vi "MoveMultiDrives.vi"(0 "Start Counter":dbl[](array[numeric]), 1 "Matched Configurations In":T2[](array[typedef]) {"Static Drive Configuration"."Indexer Mode  (FSA)" items=["Incremental", "Absolute"]; "Static Drive Configuration"."Buffer at Stop (SSH)" items=["Clear buffer", "Save and Continue"]; "Static Drive Configuration"."Buffer at Limit (SSG)" items=["Clear buffer", "Save and Continue"]; "Static Drive Configuration"."RS232 Echo Control (SSA)" items=["Echo ON", "Echo OFF"]; "Static Drive Configuration"."Reference edge of Home (OSH)" items=["CW", "CCW"]; "Static Drive Configuration"."Encoder Z for Home (OSD)" items=["Don't use", "Enable"]; "Static Drive Configuration"."Home Switch Sense (OSC)" items=["Normally Open", "Normally Closed"]; "Static Drive Configuration"."Home Position (OSB)" items=["Anywhere in Switch", "Edge of Switch"]; "Static Drive Configuration"."Limit Switch Sense (OSA)" items=["Normally Closed", "Normally Open"]; "Static Drive Configuration"."Limit Disable (LD)" items=["Both Enabled", "CW Disabled", "CCW Disabled", "Both Disabled"]; "Static Drive Configuration"."Stall Detect (FSH)" items=["Disable", "Enable"]; "Static Drive Configuration"."OP2 in Deadband (FSG)" items=["Don't Use", "ACTIVATE"]; "Static Drive Configuration"."Stop on Trigger 3 (FSF)" items=["Ignore", "STOP!"]; "Static Drive Configuration"."Activate OP1 on stall (FSE)" items=["Do not Activate", "ACTIVATE!"]; "Static Drive Configuration"."Stop on Stall (FSD)" items=["Continue", "STOP"]; "Static Drive Configuration"."Position Maintenance (FSC)" items=["Disabled", "Enabled"]; "Static Drive Configuration"."Step Mode  (FSB)" items=["Motor", "Encoder"]; "Static Drive Configuration"."Encoder Resolution (ER)" min=1 max=50000; "Static Drive Configuration"."Dead Band Window (DW)" min=0 max=999999999; "Static Drive Configuration"."Dead Band (DB)" min=0 max=999999999; "Static Drive Configuration"."Correction Gain % (CG)" items=["n/a", "12.5", "25", "37.5", "50", "62.5", "75", "87.5", "100"]; "Channel Properties"."Current Pos" format="%.2f"; "Channel Properties"."Backlash/Eng units" format="%.2f"; "Channel Properties"."Pulses/rev" format="%.2f"; "Channel Properties"."Pos Tolerance" format="%.2f"; "Channel Properties"."Pulses/unit" format="%.2f"; "Channel Properties"."Acc. Min" format="%.2f"; "Channel Properties"."Acc. Max" format="%.2f"; "Channel Properties"."Vel. Min" format="%.2f"; "Channel Properties"."Vel. Max" format="%.2f"; "Channel Properties"."Acc. Default" format="%.2f"; "Channel Properties"."Vel. Default" format="%.2f"}, 2 "GoTo Array (pulse position some channels)":T5[](array[typedef]) {"Acceleration" format="%.2f"; "Velocity" format="%.2f"; "Go To Position" step=100000.0}, 3 "Final move":bool, 4 "Predicted Move Time":dbl format="%.2f") -> (5 "Error string":string, 6 "Stop Pressed?":bool, 7 "Matched Configurations Out":T2[](array[typedef]) {"Static Drive Configuration"."Indexer Mode  (FSA)" items=["Incremental", "Absolute"]; "Static Drive Configuration"."Buffer at Stop (SSH)" items=["Clear buffer", "Save and Continue"]; "Static Drive Configuration"."Buffer at Limit (SSG)" items=["Clear buffer", "Save and Continue"]; "Static Drive Configuration"."RS232 Echo Control (SSA)" items=["Echo ON", "Echo OFF"]; "Static Drive Configuration"."Reference edge of Home (OSH)" items=["CW", "CCW"]; "Static Drive Configuration"."Encoder Z for Home (OSD)" items=["Don't use", "Enable"]; "Static Drive Configuration"."Home Switch Sense (OSC)" items=["Normally Open", "Normally Closed"]; "Static Drive Configuration"."Home Position (OSB)" items=["Anywhere in Switch", "Edge of Switch"]; "Static Drive Configuration"."Limit Switch Sense (OSA)" items=["Normally Closed", "Normally Open"]; "Static Drive Configuration"."Limit Disable (LD)" items=["Both Enabled", "CW Disabled", "CCW Disabled", "Both Disabled"]; "Static Drive Configuration"."Stall Detect (FSH)" items=["Disable", "Enable"]; "Static Drive Configuration"."OP2 in Deadband (FSG)" items=["Don't Use", "ACTIVATE"]; "Static Drive Configuration"."Stop on Trigger 3 (FSF)" items=["Ignore", "STOP!"]; "Static Drive Configuration"."Activate OP1 on stall (FSE)" items=["Do not Activate", "ACTIVATE!"]; "Static Drive Configuration"."Stop on Stall (FSD)" items=["Continue", "STOP"]; "Static Drive Configuration"."Position Maintenance (FSC)" items=["Disabled", "Enabled"]; "Static Drive Configuration"."Step Mode  (FSB)" items=["Motor", "Encoder"]; "Static Drive Configuration"."Encoder Resolution (ER)" min=1 max=50000; "Static Drive Configuration"."Dead Band Window (DW)" min=0 max=999999999; "Static Drive Configuration"."Dead Band (DB)" min=0 max=999999999; "Static Drive Configuration"."Correction Gain % (CG)" items=["n/a", "12.5", "25", "37.5", "50", "62.5", "75", "87.5", "100"]; "Channel Properties"."Current Pos" format="%.2f"; "Channel Properties"."Backlash/Eng units" format="%.2f"; "Channel Properties"."Pulses/rev" format="%.2f"; "Channel Properties"."Pos Tolerance" format="%.2f"; "Channel Properties"."Pulses/unit" format="%.2f"; "Channel Properties"."Acc. Min" format="%.2f"; "Channel Properties"."Acc. Max" format="%.2f"; "Channel Properties"."Vel. Min" format="%.2f"; "Channel Properties"."Vel. Max" format="%.2f"; "Channel Properties"."Acc. Default" format="%.2f"; "Channel Properties"."Vel. Default" format="%.2f"})   [LabVIEW 2012]
uses:
  ~subVIs/DriveClusterLower.ctl
  ~subVIs/AxisConfigCluster.ctl
  ~subVIs/DriveProperties.ctl
  ~subVIs/DriveStaticConfig.ctl
  ~subVIs/DriveStatus.ctl
  ~subVIs/GenericDriveCommand.ctl
  ~subVIs/DriveConfigGlobal.vi
  Anemometry/Anemometry Sub Vis/Globals/Trav_pos_global.vi
panel:
  out "x*y":dbl
  out "Move On Track?":bool
  out "Live Position":dbl[](array[numeric]) format="%.2f"
  out "Server copy Location":path
  out "Log File":path
  out "Move Terminated on Timeout":bool
  in  "Axis info cluster":T1
  out "Start Time":dbl format="%.2f"
  out "Running":bool
  out "Bar2":dbl(slide)=2.0 scale=-599243.8..-600063.0
  out "Bar1":dbl(slide)=2.0 scale=233922.756..233952.0
  out "Bar0":dbl(slide)=2.0 scale=322356.2..321537.0
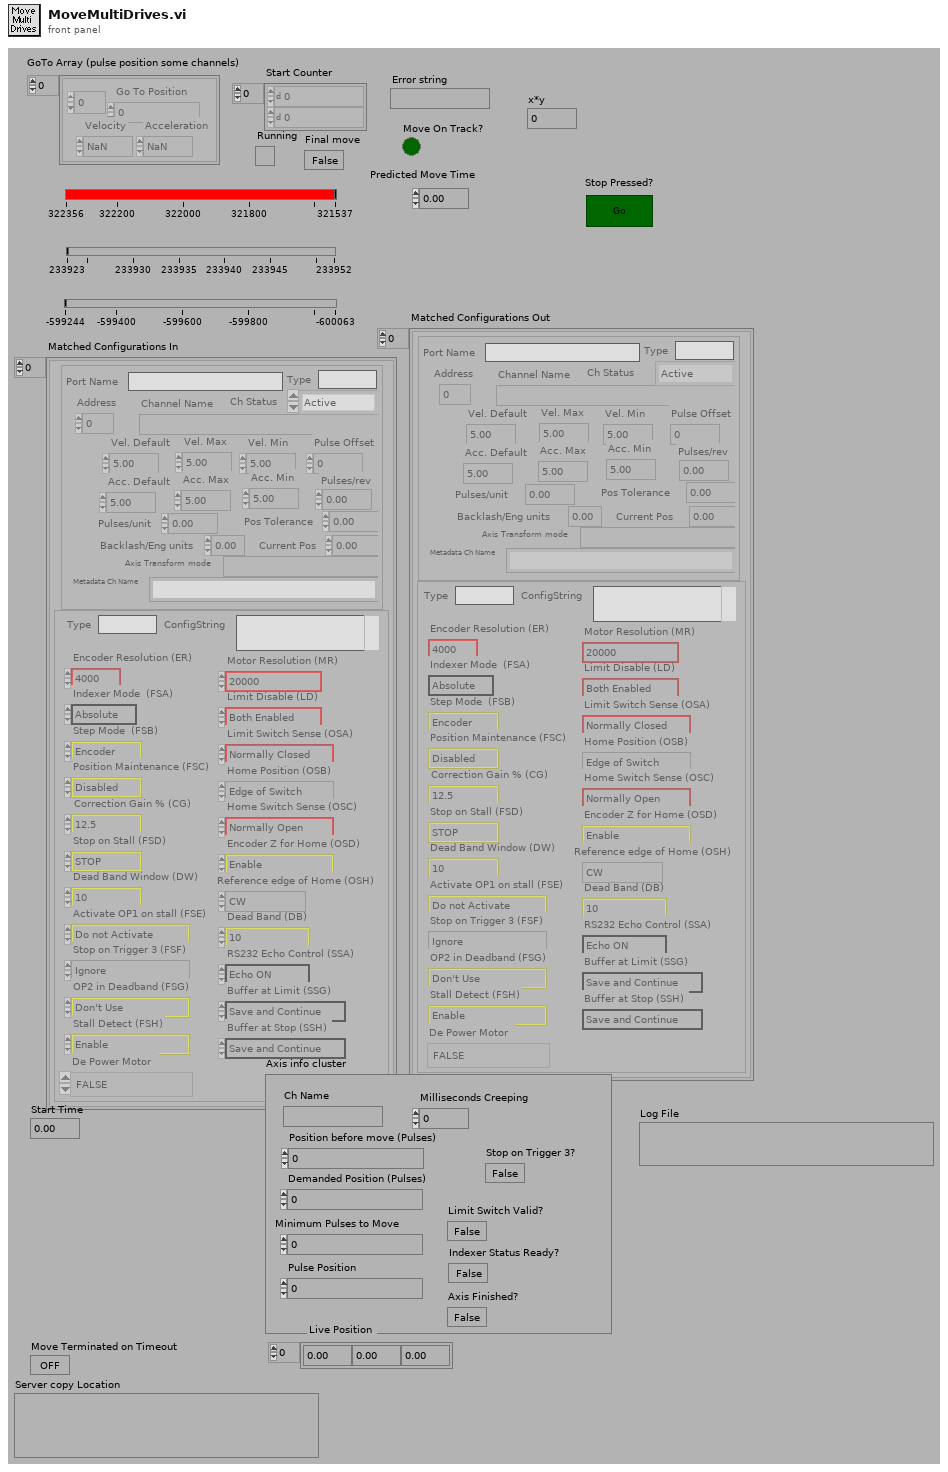
[diagram p1: front panel]
types:
  T1 = typedef "DriveStatus.ctl" = cluster{"Ch Name":string, "Position before move (Pulses)":dbl, "Demanded Position (Pulses)":dbl, "Minimum Pulses to Move":dbl, "Pulse Position":dbl, "Indexer Status Ready?":bool, "Axis Finished?":bool, "Limit Switch Valid?":bool, "Milliseconds Creeping":u32, "Stop on Trigger 3?":bool}
  T2 = typedef "AxisConfigCluster.ctl" = cluster{"Channel Properties":T3, "Static Drive Configuration":T4}
  T3 = typedef "DriveProperties.ctl" = cluster{"Channel Name":string, "Vel. Default":dbl, "Acc. Default":dbl, "Vel. Max":dbl, "Vel. Min":dbl, "Acc. Max":dbl, "Acc. Min":dbl, "Pulses/unit":dbl, "Address":u8, "Pulse Offset":i32, "Pos Tolerance":dbl, "Pulses/rev":dbl, "Backlash/Eng units":dbl, "Current Pos":dbl, "Ch Status":enum16{"Active", "Offline", "Simulate"}, "Port Name":string, "Axis Transform mode":string, "Metadata Ch Name":string, "Type":string}
  T4 = typedef "DriveStaticConfig.ctl" = cluster{"Correction Gain % (CG)":u16, "Dead Band (DB)":i32, "Dead Band Window (DW)":i32, "Encoder Resolution (ER)":i32, "Step Mode  (FSB)":u16, "Position Maintenance (FSC)":u16, "Stop on Stall (FSD)":u16, "Activate OP1 on stall (FSE)":u16, "Stop on Trigger 3 (FSF)":u16, "OP2 in Deadband (FSG)":u16, "Stall Detect (FSH)":u16, "Limit Disable (LD)":u16, "Motor Resolution (MR)":enum16{"200", "400", "1000", "2000", "4000", "5000", "10000", "12800", "18000", "20000", "21600", "25000", "25400", "25600", "36000", "50000", "278528", "425984", "507904", "614400", "655360", "819200", "1024000"}, "Limit Switch Sense (OSA)":u16, "Home Position (OSB)":u16, "Home Switch Sense (OSC)":u16, "Encoder Z for Home (OSD)":u16, "Reference edge of Home (OSH)":u16, "RS232 Echo Control (SSA)":u16, "Buffer at Limit (SSG)":u16, "Buffer at Stop (SSH)":u16, "Indexer Mode  (FSA)":u16, "Type":string, "ConfigString":string, "De Power Motor":enum16{"TRUE", "FALSE"}}
  T5 = typedef "DriveClusterLower.ctl" = cluster{"Go To Position":dbl, "Velocity":dbl, "Acceleration":dbl, "Address":u8}
  T6 = typedef "GenericDriveCommand.ctl" = string
  T7 = cluster{"GenericDriveCommand":T6, "Go To Position":dbl}
  T8 = cluster{"GenericDriveCommand":T6, "Acceleration":dbl}
  T9 = cluster{"GenericDriveCommand":T6, "Acceleration":dbl}[]
  T10 = enum16{"A-    Acceleration (rps)", "B-    Buffer Status", "C-    Continue", "CG-  Correction Gain", "CR-  Cariage Return", "D-    Distance (pulses)", "DB-  Dead Band (encoder steps)", "DW- Deadband Window (encoder steps)", "E-    Enable Communications", "ER-  Encoder Resolution (steps/rev)", "F-    Disable Communications", "FS-  Encoder Functions Report", "FSA- Incremental/Absolute (0/1)", "FSB- Motor/Encoder Step Mode (0/1)", "FSC- Enable/Disable Position Maint. (1/0)", "FSD- Stop/Continue on Stall (1/0)", "FSE- Activate o/p1 on Stall (1/0)", "FSF- Stop Motion on Trig3 (1/0)", "FSG- Activate o/p2 in Deadband (1/0)", "FSH- Enable Stall Detect (1/0)", "G- Go", "GH- Go Home and Zero (+/-V)", "^H- Delete ", "H- Direction Reverse/CCW/CW (0,1,2)", "IS- Input Status", "K- Kill", "L- Loop (n)", "LD- Limit DISABLE (0-none,1-CW,2-CCW,3-Both)", "LF- Line Feed", "MC- Mode Continuous", "MN- Mode Normal", "MPA- Motor Postion Absolute", "MPI- Motor Position Incremental", "MR- Motor Resolution (Drive Steps/rev)", "N- End of Loop", "O- Output (00,01,10,11)", "OS- Report Homing Setup", "OSA- NO/NC Limits (1/0)", "OSB- Back Up to Home/Edge? (0/1)", "OSC- NO/NC Home Switch (1/0)", "OSD- Enable Encoder Z for Home (0/1)", "OSH- Reference Edge for Home CW/CCW (0/1)", "PR- Report ABSOLUTE Position", "PS- Pause until Continue", "PX- Report Absolute ENCODER Position", "PZ- Zero Absolute Counter", "\"- Quote (17 ASCII +Space)", "Q- Enter/Exit Velocity Profiling (1/0)", "R- Request Indexer Status", "RA- Report Limit Switch Status", "RB- Report Loop, Pause, Shutdown, Trigger Status", "RC- Report Closed Loop Status", "RM- Velocity Streaming Rate Multiplier (000-FFF)", "RV- Report Revision Level", "S- Controlled Stop", "SN- Debounce (1-1000ms)", "SS- Report Software Switch Status", "SSA- Disable RS232 Echo (1/0)", "SSG- Clear/Save Command Buffer on Limit (0/1)", "SSH- Clear/Save Command Buffer on Stop (0/1)", "ST- Shutdown (1/0)", "SV- Servoing Setting (0,1,2,3)", "T- Time Delay (0.01-99999.99)", "TR- Wait for Trigger High/Low/Ignore (1/0/X)", "TS- Report Trigger Status", "U- Pause after Move Until Continue", "V- Velocity (0.01-50.00 revs/sec)", "W1- Report Relative Position <Signed Binary>", "W3- Report Relative Position <Hexadecimal>", "Y- Abort Loop at N", "Z-    Reset to Defaults", "#-    Disable/Set Soft Addresses (0/1-255)"}
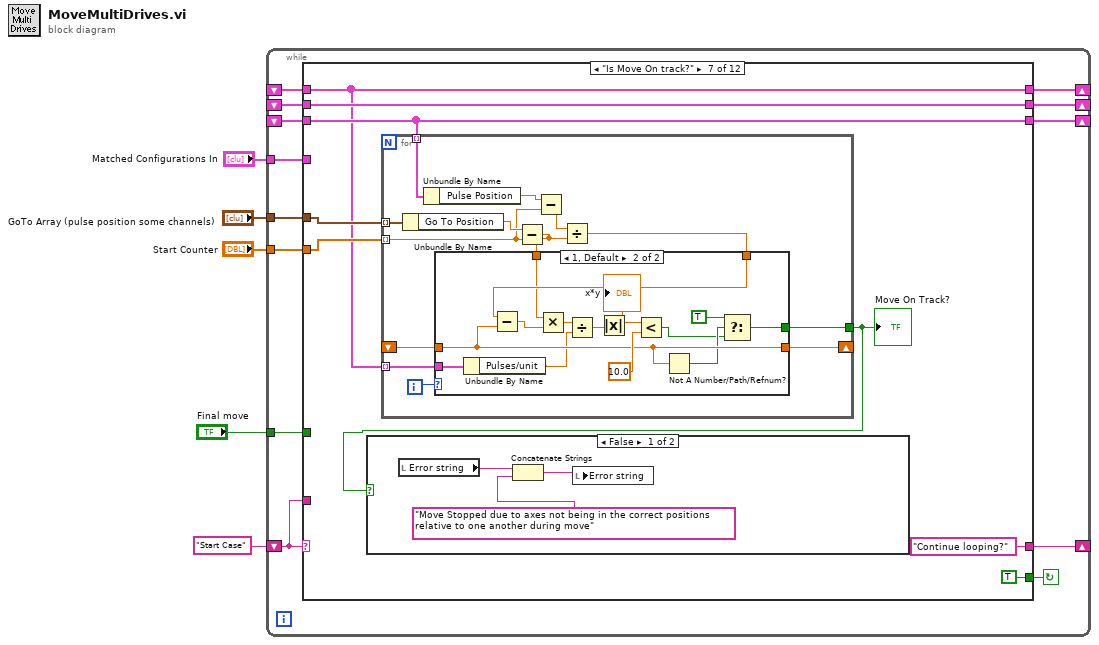
[diagram p0: block diagram]
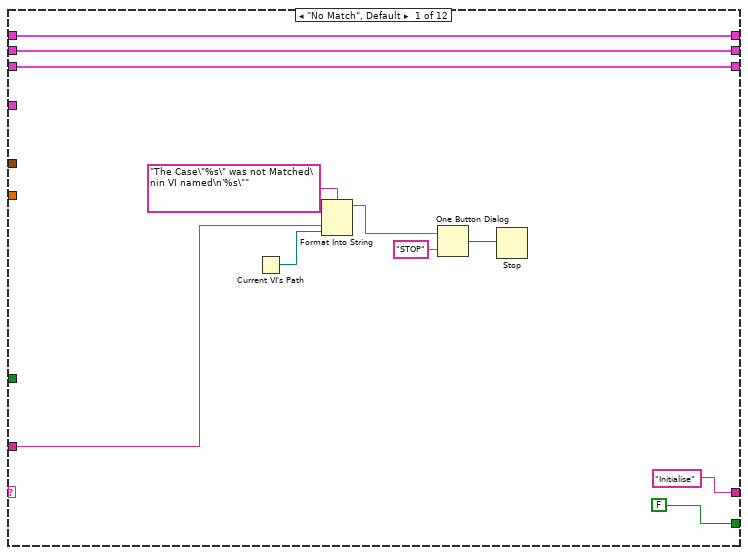
[diagram p2: hidden frame]
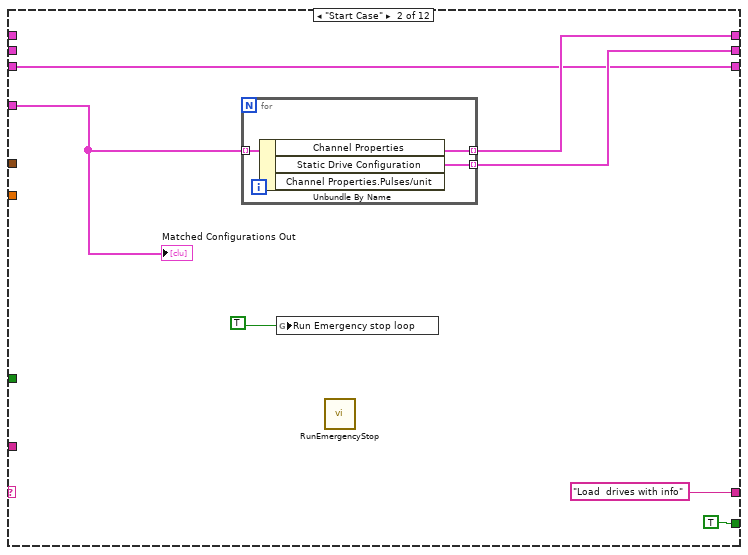
[diagram p3: hidden frame]
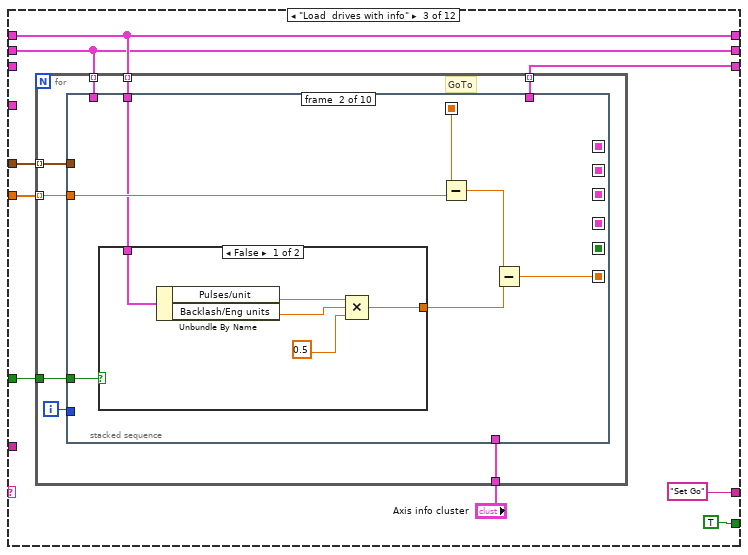
[diagram p4: hidden frame]
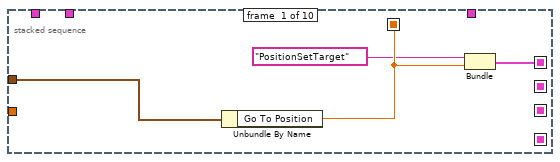
[diagram p5: hidden frame]
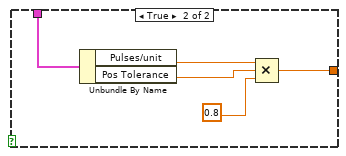
[diagram p6: hidden frame]
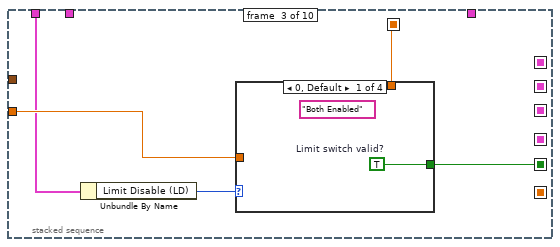
[diagram p7: hidden frame]
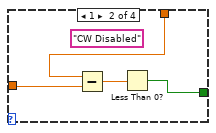
[diagram p8: hidden frame]
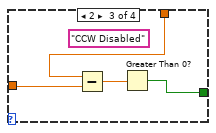
[diagram p9: hidden frame]
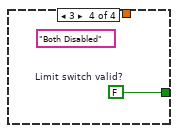
[diagram p10: hidden frame]
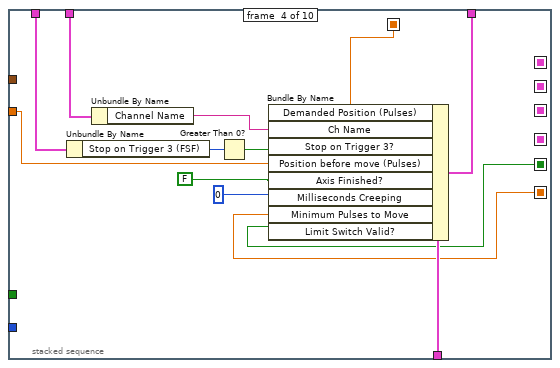
[diagram p11: hidden frame]
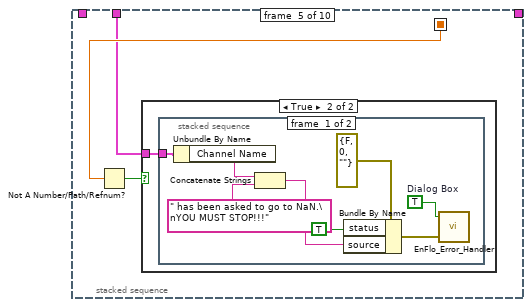
[diagram p12: hidden frame]
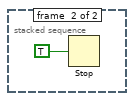
[diagram p14: hidden frame]
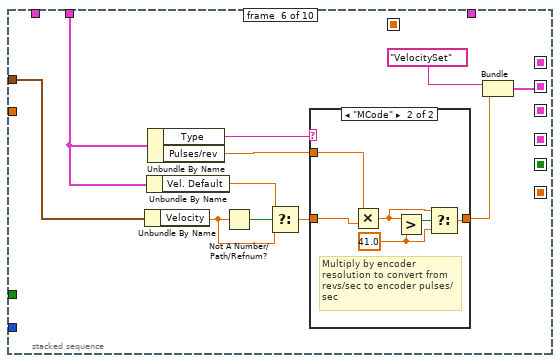
[diagram p15: hidden frame]
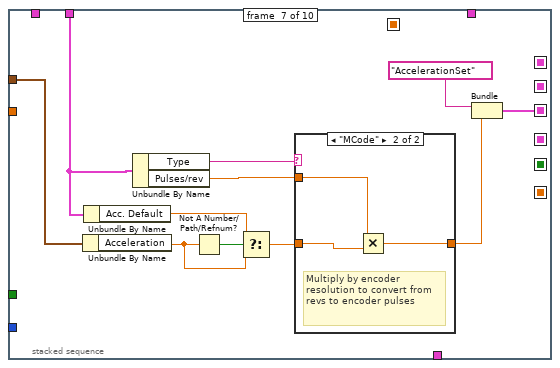
[diagram p17: hidden frame]
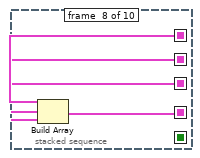
[diagram p19: hidden frame]
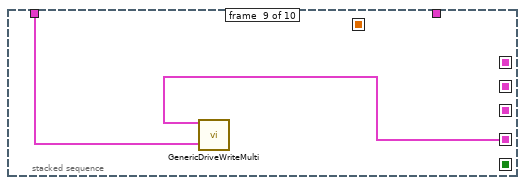
[diagram p20: hidden frame]
diagram:
  n1 = while {
    shift-left: _ -> [w7]
    shift-right: [w6] -> _
    tunnel: "Final move" -> [w8]
    tunnel: "Start Counter" -> [w9]
    tunnel: "GoTo Array (pulse position some channels)" -> [w10]
    tunnel: "Matched Configurations In" -> [w15]
    shift-left: _ -> [w11]
    shift-right: [w13] -> _
    shift-left: _ -> [w12]
    shift-right: [w14] -> _
    shift-left: "Start Case" -> [w16]
    shift-right: [w17] -> _
    stop <- w18 continue-if-true
    n2 = case shown="\"Is Move On track?\"" w16 {
      tunnel: [FALSE TRUE TRUE TRUE TRUE TRUE TRUE TRUE TRUE TRUE TRUE FALSE] -> w18
      tunnel: ["Initialise" "Load  drives with info" "Set Go" "Record Time" "Check status of axis" "Is Move On track?" "Continue looping?" w299 "Does Log file Exist" w345 "Write to Log file" "End"] -> w17
      tunnel: w16 -> [w24 _ _ _ _ _ _ _ _ _ _ _]
      tunnel: w15 -> [_ w30 _ w181 _ _ _ _ _ _ _ _]
      tunnel: [w21 w33 w45 w185 w196 w203 w256 w318 w326 w350 w371 w398] -> w14
      tunnel: [w20 w32 w42 w184 w195 w204 w261 w317 w325 w349 w370 w397] -> w13
      tunnel: w12 -> [w21 _ w45 w185 w196 w203 w256 w318 w326 w350 w371 w398]
      tunnel: w11 -> [w20 _ w42 w184 w195 w204 w261 w317 w325 w349 w370 w397]
      tunnel: w10 -> [_ _ w46 _ _ _ w263 _ _ _ _ _]
      tunnel: w9 -> [_ _ w44 _ _ _ w262 _ _ _ _ _]
      tunnel: w8 -> [_ _ w43 _ _ _ _ _ _ _ _ _]
      tunnel: [w19 w31 w40 w182 w193 w200 w260 w304 w324 w348 w369 w395] -> w6
      tunnel: w7 -> [w19 w31 _ w182 w193 w201 w260 w304 w324 w348 w369 w395]
      frame "No Match", Default {
        n3 = Current VI's Path() -> (path=w23:path)
        n4 = Format Into String(format string="The Case\"%s\" was not Matched\nin VI named\n'%s\"" ("Format String"), w24, w23) -> (resulting string=w27:string)  [unwired: 2 in, 1 out]
        n5 = One Button Dialog(message=w27, button name ("OK")="STOP") -> (true=w25:bool)
        n6 = Stop(stop? (T)=w25) -> ()
      }
      frame "Start Case" {
        n7 = for {
          tunnel: w30 -> [w39] mode=indexing
          tunnel: [w38] -> w33 mode=indexing
          tunnel: [w37] -> w32 mode=indexing
          n8 = Unbundle By Name(w39) -> ("Channel Properties"=w38:T3, "Static Drive Configuration"=w37:T4)  [unwired: 1 out]
        }
        n9 = global write "DriveConfigGlobal.vi" "Run Emergency stop loop"(TRUE) -> ()
        n10 = call "RunEmergencyStop.vi"() -> ()  [unwired: 1 in, 7 out]
        "Matched Configurations Out" <- w30
      }
      frame "Load  drives with info" {
        n11 = for {
          tunnel: w46 -> [w55] mode=indexing
          tunnel: w45 -> [w54] mode=indexing
          tunnel: w44 -> [w53] mode=indexing
          tunnel: w43 -> [w52]
          tunnel: w42 -> [w51] mode=indexing
          tunnel: "Axis info cluster" -> [w50]
          tunnel: [w49] -> w40 mode=indexing
          i -> [w56]
          # "GoTo"
          n12 = stacked-sequence {
            seq-local: [w59 _ _ _ _ _ _ _ _ _] -> [_ w67 w81 w96 w108 _ _ _ _ w163]
            seq-local: [w58 _ _ _ _ _ _ _ _ _] -> [_ _ _ _ _ _ _ w155 _ _]
            seq-local: [_ _ _ _ _ w125 _ _ _ _] -> [_ _ _ _ _ _ _ w154 _ _]
            seq-local: [_ _ _ _ _ _ w143 _ _ _] -> [_ _ _ _ _ _ _ w153 _ _]
            seq-local: [_ _ _ _ _ _ _ w152 _ _] -> [_ _ _ _ _ _ _ _ w157 _]
            seq-local: [_ w62 _ _ _ _ _ _ _ _] -> [_ _ _ w103 _ _ _ _ _ _]
            seq-local: [_ _ w78 _ _ _ _ _ _ _] -> [_ _ _ w101 _ _ _ _ _ _]
            tunnel: w55 -> [w60 _ _ _ _ w129 w147 _ _ _]
            tunnel: w56 -> [_ _ _ _ _ _ _ _ _ w164]
            tunnel: w52 -> [_ w65 _ _ _ _ _ _ _ _]
            tunnel: w54 -> [_ w63 _ w105 w106 w123 w141 _ w156 _]
            tunnel: w53 -> [_ w64 w80 w98 _ _ _ _ _ w162]
            tunnel: w51 -> [_ _ w79 w100 _ _ _ _ _ _]
            tunnel: w50 -> [_ _ _ w104 _ _ _ _ _ _]
            tunnel: [_ _ _ w102 _ _ _ _ _ _] -> w49
            frame #0 {
              n13 = Unbundle By Name(w60) -> ("Go To Position"=w59:dbl)
              n14 = Bundle("GenericDriveCommand"=T6 "PositionSetTarget", "Go To Position"=w59) -> (w58:T7)  [unwired: 1 out]
            }
            frame #1 {
              n15 = case shown="False" w65 {
                tunnel: w63 -> [w72 w77]
                tunnel: [w68 w73] -> w66
                frame False {
                  n16 = Unbundle By Name(w72) -> ("Pulses/unit"=w71:dbl, "Backlash/Eng units"=w70:dbl)
                  n17 = Compound Arithmetic op=MULTIPLY(w71, w70, 0.5) -> (w68:dbl)
                }
                frame True {
                  n18 = Unbundle By Name(w77) -> ("Pulses/unit"=w76:dbl, "Pos Tolerance"=w75:dbl)
                  n19 = Compound Arithmetic op=MULTIPLY(w76, w75, 0.8) -> (w73:dbl)
                }
              }
              n20 = Subtract(x=w67, y=w64) -> (x-y=w61:dbl)
              n21 = Subtract(x=w61, y=w66) -> (x-y=w62:dbl)
            }
            frame #2 {
              n22 = Unbundle By Name(w79) -> ("Limit Disable (LD)"=w82:u16)
              n23 = case shown="0, Default" w82 {
                tunnel: [w83 w84 w88 w92] -> w78
                tunnel: w80 -> [_ w86 w90 _]
                tunnel: w81 -> [_ w87 w91 _]
                frame 0, Default {
                  w83 = TRUE  # Limit switch valid?
                  (unwired) "Both Enabled"
                }
                frame 1 {
                  (unwired) "CW Disabled"
                  n24 = Subtract(x=w87, y=w86) -> (x-y=w85:dbl)
                  n25 = Less Than 0?(x=w85) -> (x < 0?=w84:bool)
                }
                frame 2 {
                  (unwired) "CCW Disabled"
                  n26 = Subtract(x=w91, y=w90) -> (x-y=w89:dbl)
                  n27 = Greater Than 0?(x=w89) -> (x > 0?=w88:bool)
                }
                frame 3 {
                  (unwired) "Both Disabled"
                  w92 = FALSE  # Limit switch valid?
                }
              }
            }
            frame #3 {
              n28 = Unbundle By Name(w100) -> ("Stop on Trigger 3 (FSF)"=w99:u16)
              n29 = Unbundle By Name(w105) -> ("Channel Name"=w97:string)
              n30 = Greater Than 0?(x=w99) -> (x > 0?=w95:bool)
              n31 = Bundle By Name(cluster=w104, "Demanded Position (Pulses)"=w96, "Ch Name"=w97, "Stop on Trigger 3?"=w95, "Position before move (Pulses)"=w98, "Axis Finished?"=FALSE ("Bundle Element"), "Milliseconds Creeping"=u32 0 ("Bundle Element"), "Minimum Pulses to Move"=w103, "Limit Switch Valid?"=w101) -> (w102:T1)
            }
            frame #4 {
              n32 = Not A Number/Path/Refnum?(number/path/refnum=w108) -> (NaN/Path/Refnum?=w107:bool)
              n33 = case shown="True" w107 {
                tunnel: w106 -> [_ w109]
                frame False {
                }
                frame True {
                  n34 = stacked-sequence {
                    tunnel: w109 -> [w117 _]
                    frame #0 {
                      w110 = TRUE  # Dialog Box
                      n35 = Unbundle By Name(w117) -> ("Channel Name"=w113:string)
                      n36 = Concatenate Strings(w113, " has been asked to go to NaN.\nYOU MUST STOP!!!") -> (w111:string)
                      n37 = Bundle By Name(cluster=errorcluster {"status"=FALSE, "code"=0, "source"=""} ("error in (no error)"), "status"=TRUE ("Bundle Element"), "source"=w111) -> (w115:errorcluster)
                      n38 = call "EnFlo_Error_Handler.vi"("error in (no error)"=w115, "Dialog Box (T)"=w110) -> ()  [unwired: 1 in, 3 out]
                    }
                    frame #1 {
                      n39 = Stop(stop? (T)=TRUE) -> ()
                    }
                  }
                }
              }
            }
            frame #5 {
              n40 = Unbundle By Name(w129) -> ("Velocity"=w126:dbl)
              n41 = Unbundle By Name(w123) -> ("Vel. Default"=w127:dbl)
              n42 = Unbundle By Name(w123) -> ("Type"=w122:string, "Pulses/rev"=w120:dbl)
              n43 = Not A Number/Path/Refnum?(number/path/refnum=w126) -> (NaN/Path/Refnum?=w128:bool)
              n44 = Select(t=w127, s=w128, f=w126) -> (s? t:f=w121:dbl)
              n45 = case shown="\"MCode\"" w122 {
                tunnel: w121 -> [w130 w131]
                tunnel: w120 -> [_ w136]
                tunnel: [w130 w135] -> w119
                frame "ParkerX", Default {
                }
                frame "MCode" {
                  w132 = 41.0 ("y")
                  # "Multiply by encoder resolution to convert from revs/sec to encoder pulses/sec"
                  n46 = Multiply(x=w136, y=w131) -> (x*y=w133:dbl)
                  n47 = Greater?(x=w133, y=w132) -> (0:w134:bool)
                  n48 = Select(t=w133, s=w134, f=w132) -> (s? t:f=w135:dbl)
                }
              }
              n49 = Bundle("GenericDriveCommand"=T6 "VelocitySet", "y"=w119) -> (w125:cluster{"GenericDriveCommand":T6, "y":dbl})  [unwired: 1 out]
            }
            frame #6 {
              n50 = Unbundle By Name(w147) -> ("Acceleration"=w144:dbl)
              n51 = Unbundle By Name(w141) -> ("Acc. Default"=w145:dbl)
              n52 = Unbundle By Name(w141) -> ("Type"=w140:string, "Pulses/rev"=w139:dbl)
              n53 = Not A Number/Path/Refnum?(number/path/refnum=w144) -> (NaN/Path/Refnum?=w146:bool)
              n54 = Select(t=w145, s=w146, f=w144) -> (s? t:f=w138:dbl)
              n55 = case shown="\"MCode\"" w140 {
                tunnel: w138 -> [w148 w151]
                tunnel: w139 -> [_ w150]
                tunnel: [w148 w149] -> w137
                frame "ParkerX", Default {
                }
                frame "MCode" {
                  # "Multiply by encoder resolution to convert from revs to encoder pulses"
                  n56 = Multiply(x=w150, y=w151) -> (x*y=w149:dbl)
                }
              }
              n57 = Bundle("GenericDriveCommand"=T6 "AccelerationSet", "Acceleration"=w137) -> (w143:T8)  [unwired: 1 out]
            }
            frame #7 {
              n58 = Build Array(w155, w154, w153) -> (w152:T9)
            }
            frame #8 {
              n59 = call "GenericDriveWriteMulti.vi"("Channel Description"=w156, "Array Constant"=w157) -> ()  [unwired: 1 out]
            }
            frame #9 {
              n60 = Less?(x=w163, y=w162) -> (x < y?=w161:bool)
              n61 = Max & Min(x=w163, y=w162) -> (max(x,y)=w166:dbl, min(x,y)=w165:dbl)
              n62 = Select(t=2, s=w161, f=1 ("Fill Style")) -> (s? t:f=w158:i32)
              n63 = case shown="1" w164 {
                tunnel: w166 -> [w170 w174 w178]
                tunnel: w165 -> [w169 w173 w177]
                tunnel: w161 -> [w168 w172 w176]
                tunnel: w158 -> [w167 w171 w175]
                frame 0, Default {
                  n64 = property on="Bar0" class="Slide (strict)"("Scale.Range:Maximum"=w170, "Scale.Range:Minimum"=w169, "Scale.Flipped"=w168, "Fill Style"=w167) -> ()  [unwired: 2 in, 2 out]
                }
                frame 1 {
                  n65 = property on="Bar1" class="Slide (strict)"("Scale.Range:Maximum"=w174, "Scale.Range:Minimum"=w173, "Scale.Flipped"=w172, "Fill Style"=w171) -> ()  [unwired: 2 in, 2 out]
                }
                frame 2 {
                  n66 = property on="Bar2" class="Slide (strict)"("Scale.Range:Maximum"=w178, "Scale.Range:Minimum"=w177, "Scale.Flipped"=w176, "Fill Style"=w175) -> ()  [unwired: 2 in, 2 out]
                }
              }
            }
          }
        }
      }
      frame "Set Go" {
        n67 = call "GetActivePortNames.vi"("Matched Configurations In"=w181) -> ("Port Name Array"=w180:string[], "Drive Type Array"=w179:string[])
        n68 = for {
          tunnel: w180 -> [w191] mode=indexing
          tunnel: "Global" -> [w190]
          tunnel: w179 -> [w189] mode=indexing
          n69 = call "GenericDriveIO.vi"("GenericDriveCommand"=T6 "GoNow", "Channel Name"=w190, "Type"=w189, "Port Name"=w191) -> ()  [unwired: 2 in, 6 out]
        }
      }
      frame "Record Time" {
        n70 = Get Date/Time In Seconds() -> (seconds since 1Jan1904=w192:timestamp)
        n71 = To Double Precision Float(number=w192) -> (double precision float=→"Start Time":dbl)
      }
      frame "Check status of axis" {
        (unwired) "Global"
        n72 = for {
          shift-right: [w210] -> w199
          shift-left: "" -> [w212]
          tunnel: w203 -> [w211] mode=indexing
          tunnel: w201 -> [w208] mode=indexing
          tunnel: [w207] -> w200 mode=indexing
          i -> [w213]
          n73 = Unbundle By Name(w208) -> ("Axis Finished?"=w209:bool)
          n74 = case shown="False" w209 {
            tunnel: w213 -> [w235 _]
            tunnel: w212 -> [w234 w255]
            tunnel: w211 -> [w229 _]
            tunnel: [w232 w255] -> w210
            tunnel: w208 -> [w231 w254]
            tunnel: [w230 w254] -> w207
            frame False {
              n75 = Unbundle By Name(w229) -> ("Channel Name"=w224:string, "Pulses/unit"=w228:dbl, "Pulse Offset"=w225:i32)
              n76 = call "CheckDriveStatus.vi"("Channel Properties"=w229, "Axis info cluster"=w231) -> ("Error string"=w233:string, "Axis info cluster Out"=w230:T1)
              n77 = Unbundle By Name(w230) -> ("Pulse Position"=w214:dbl)
              n78 = global read "Trav_pos_global.vi" "Live Position"() -> (w216:dbl[])
              n79 = Match Pattern(string=w224, regular expression=":") -> (before substring=w220:string, after substring=w219:string)  [unwired: 1 in, 2 out]
              n80 = Match Pattern(string=w219, regular expression=":") -> (after substring=w218:string)  [unwired: 1 in, 3 out]
              n81 = Add(x=w225, y=w214) -> (x+y=w226:dbl)
              n82 = Divide(x=w226, y=w228) -> (x/y=w217:dbl)
              n83 = case shown="\"Z\", Default" w218 {
                tunnel: w217 -> [w237 w242 w250]
                tunnel: w216 -> [w239 w245 w249]
                tunnel: [w236 w241 w246] -> w215
                frame "Y" {
                  n84 = Index Array(array=w239) -> (element #1=w238:dbl, element #3=w240:dbl)  [unwired: 3 in, 1 out]
                  n85 = Build Array(w238, w237, w240) -> (w236:dbl[])
                }
                frame "X" {
                  n86 = Index Array(array=w245) -> (element #2=w243:dbl, element #3=w244:dbl)  [unwired: 3 in, 1 out]
                  n87 = Build Array(w242, w243, w244) -> (w241:dbl[])
                }
                frame "Z", Default {
                  n88 = Index Array(array=w249) -> (element #1=w248:dbl, element #2=w247:dbl)  [unwired: 2 in]
                  n89 = Build Array(w248, w247, w250) -> (w246:dbl[])
                }
              }
              n90 = call "Coordinate_transforms.vi"("Traverse Name"=w220, "Input"=w215, "Mode"=enum16{"XYZ to Channel", "Channel to XYZ"}."Channel to XYZ") -> ("Output"=w222:dbl[])
              "Live Position" <- w222
              n91 = Concatenate Strings(w234, w233) -> (w232:string)
              n92 = case shown="2" w235 {
                tunnel: w214 -> [w251 w252 w253]
                frame 0, Default {
                  "Bar0" <- w251
                }
                frame 1 {
                  "Bar1" <- w252
                }
                frame 2 {
                  "Bar2" <- w253
                }
              }
              n93 = global write "Trav_pos_global.vi" "Live Position"(w222) -> ()
            }
            frame True {
            }
          }
        }
        "Error string" <- w199
      }
      frame "Is Move On track?" {
        n94 = for {
          tunnel: w260 -> [w279] mode=indexing
          tunnel: w263 -> [w278] mode=indexing
          tunnel: w262 -> [w275] mode=indexing
          shift-right: [w271] -> _
          shift-left: _ -> [w272]
          tunnel: [w268] -> w257
          tunnel: w256 -> [w267] mode=indexing
          i -> [w273]
          n95 = Unbundle By Name(w278) -> ("Go To Position"=w277:dbl)
          n96 = Unbundle By Name(w279) -> ("Pulse Position"=w276:dbl)
          n97 = Subtract(x=w277, y=w275) -> (x-y=w269:dbl)
          n98 = Subtract(x=w276, y=w275) -> (x-y=w274:dbl)
          n99 = Divide(x=w274, y=w269) -> (x/y=w270:dbl)
          n100 = case shown="1, Default" w273 {
            tunnel: [w281 w291] -> w271
            tunnel: w272 -> [_ w291]
            tunnel: w270 -> [w281 w295]
            tunnel: w269 -> [_ w293]
            tunnel: [TRUE w288] -> w268
            tunnel: w267 -> [_ w283]
            frame 0 {
            }
            frame 1, Default {
              n101 = Unbundle By Name(w283) -> ("Pulses/unit"=w284:dbl)
              n102 = Subtract(x=w295, y=w291) -> (x-y=w294:dbl)
              n103 = Multiply(x=w293, y=w294) -> (x*y=w285:dbl)
              n104 = Divide(x=w285, y=w284) -> (x/y=w282:dbl)
              n105 = Absolute Value(x=w282) -> (abs(x)=w286:dbl)
              "x*y" <- w286
              n106 = Less?(x=w286, y=10.0) -> (x < y?=w289:bool)
              n107 = Not A Number/Path/Refnum?(number/path/refnum=w291) -> (NaN/Path/Refnum?=w290:bool)
              n108 = Select(t=TRUE, s=w290, f=w289) -> (s? t:f=w288:bool)
            }
          }
        }
        "Move On Track?" <- w257
        n109 = case shown="False" w257 {
          frame False {
            n110 = local read "Error string"() -> (w266:string)
            n111 = Concatenate Strings(w266, "Move Stopped due to axes not being in the correct positions relative to one another during move") -> (w264:string)
            n112 = local write "Error string"(w264) -> ()
          }
          frame True {
          }
        }
      }
      frame "Continue looping?" {
        n113 = for {
          tunnel: w304 -> [w321] mode=indexing
          tunnel: [w320] -> w303 mode=indexing
          n114 = Unbundle By Name(w321) -> ("Axis Finished?"=w320:bool)
        }
        n115 = Multiply(x="Predicted Move Time", y=1.1) -> (x*y=w310:dbl)
        n116 = Add(x=w310, y=10.0) -> (x+y=w306:dbl)
        n117 = local read "Start Time"() -> (w305:dbl)
        n118 = Get Date/Time In Seconds() -> (seconds since 1Jan1904=w296:timestamp)
        n119 = To Double Precision Float(number=w296) -> (double precision float=w311:dbl)
        n120 = Subtract(x=w311, y=w305) -> (x-y=w312:dbl)
        n121 = global read "DriveConfigGlobal.vi" "Stop Pressed?"() -> (w313:bool)
        "Stop Pressed?" <- w313
        n122 = local read "Error string"() -> (w314:string)
        n123 = Less?(x=w312, y=w306) -> (x < y?=w298:bool)
        n124 = And Array Elements(Boolean array=w303) -> (logical AND=w316:bool)
        n125 = Not(x=w298) -> (.not. x?=→"Move Terminated on Timeout":bool)
        n126 = Empty String/Path?(string/path=w314) -> (empty?=w315:bool)
        n127 = Compound Arithmetic op=AND(w315, invert w316, invert w313, w298) -> (w302:bool)
        n128 = call "Program_Active.vi"() -> ()  [unwired: 1 in]
        n129 = Select(t="Check status of axis", s=w302, f="Kill All Axes") -> (s? t:f=w299:string)
      }
      frame "Kill All Axes" {
        # "Kill All Axis in case they are creeping"
        n130 = stacked-sequence {
          frame #0 {
            n131 = global read "DriveConfigGlobal.vi" "Configurations"() -> (w331:T2[])
            n132 = call "GetActivePortNames.vi"("Matched Configurations In"=w331) -> ("Port Name Array"=w330:string[], "Drive Type Array"=w328:string[])
            n133 = for {
              tunnel: w330 -> [w335] mode=indexing
              tunnel: "Global" -> [w334]
              tunnel: w328 -> [w333] mode=indexing
              (unwired) T10."K- Kill" ("COMMAND")
              n134 = call "GenericDriveIO.vi"("GenericDriveCommand"=T6 "StopEmergency", "Channel Name"=w334, "Type"=w333, "Port Name"=w335) -> ()  [unwired: 2 in, 6 out]
            }
          }
          frame #1 {
            n135 = disable-structure shown="Disabled" {
              frame Disabled {
                n136 = local read "Error string"() -> (w337:string)
                n137 = Empty String/Path?(string/path=w337) -> (empty?=w336:bool)
                n138 = case shown="False" w336 {
                  frame False {
                    n139 = call "Wait_Seconds_with_display.vi"("Message"="Traverse Stopping", "Seconds to wait"=10.0) -> ()  [unwired: 1 in, 1 out]
                  }
                  frame True {
                  }
                }
              }
              frame Enabled {
              }
            }
          }
        }
        "Running" <- FALSE
      }
      frame "Does Log file Exist" {
        n140 = call "Create_Error_log_folders.vi"("Per Day Log File?"=TRUE, "Log Filename"="Traverse_Low" ("Input Element")) -> ("exists?"=w342:bool, "Server copy Location"=→"Server copy Location":path, "Local Log File"=→"Log File":path)  [unwired: 1 in]
        n141 = Select(t="Write to Log file", s=w342, f="Create Log file") -> (s? t:f=w345:string)
      }
      frame "Create Log file" {
        n142 = Build Array("Date::", "Time::", "Seconds:Since:1st Jan 1904", "Move:Duration:Seconds", "Move:Terminated:On Timeout") -> (w360:string[])
        n143 = for {
          N: 3 -> [_]
          shift-right: [w373] -> w359
          shift-left: w360 -> [w374]
          i -> [w379]
          n144 = Increment(x=w379) -> (x+1=w378:i32)
          n145 = Number To Decimal String(number=w378) -> (decimal integer string=w377:string)  [unwired: 1 out]
          n146 = Build Array("Axis:Ch Name:", "Position Before:Move (Pulses):", "Demanded:Position (Pulses):", "Minimum Pulses:to Move:", "Pulses:Moved:", "Indexer:Status Ready:", "Axis:Finished?", "Limit:Switch Valid?") -> (w376:string[])
          n147 = for {
            tunnel: w377 -> [w390]
            tunnel: w376 -> [w389] mode=indexing
            tunnel: [w388] -> w375 mode=indexing
            n148 = Concatenate Strings(w389, w390) -> (w388:string)
          }
          n149 = Build Array (concatenate)(w374, w375) -> (w373:string[])
        }
        n150 = for {
          tunnel: w359 -> [w394] mode=indexing
          tunnel: [w393] -> w363 mode=indexing
          tunnel: [w392] -> w364 mode=indexing
          tunnel: [w391] -> w365 mode=indexing
          n151 = call "Split_Ch_name.vi"("Ch name"=w394) -> ("Top level"=w393:string, "Middle"=w392:string, "Low level"=w391:string)
        }
        n152 = local read "Log File"() -> (w352:path)
        n153 = Build Array(w363, w364, w365) -> (w361:string[][])
        n154 = Array To Spreadsheet String(array=w361, 3:"%s" ("format string")) -> (spreadsheet string=w353:string)  [unwired: 1 out]
        n155 = call "Write_File_Simple.vi"("append to file? (new file:F)"=TRUE, "character string"=w353, "file path"=w352) -> ()  [unwired: 2 out]
      }
      frame "Write to Log file" {
        n156 = stacked-sequence {
          seq-local: [w404 _ _] -> [_ w416 _]
          seq-local: [_ w415 _] -> [_ _ w442]
          tunnel: w395 -> [_ w417 _]
          frame #0 {
            n157 = local read "Move Terminated on Timeout"() -> (w411:bool)
            n158 = Get Date/Time In Seconds() -> (seconds since 1Jan1904=w403:timestamp)
            n159 = local read "Start Time"() -> (w413:dbl)
            n160 = To Double Precision Float(number=w403) -> (double precision float=w402:dbl)
            n161 = Subtract(x=w402, y=w413) -> (x-y=w412:dbl)
            n162 = Get Date/Time String(date format (0)=enum16{"short", "long", "abbreviated"}."abbreviated", seconds (now)=w403) -> (date string=w408:string, time string=w407:string)  [unwired: 1 out]
            n163 = Number To Fractional String(number=w402, precision (6)=i16 3) -> (F-format string=w400:string)  [unwired: 2 out]
            n164 = Number To Decimal String(number=w412) -> (decimal integer string=w406:string)  [unwired: 1 out]
            n165 = Select(t="TRUE", s=w411, f="FALSE") -> (s? t:f=w405:string)
            n166 = Build Array(w408, w407, w400, w406, w405) -> (w404:string[])
          }
          frame #1 {
            n167 = for {
              tunnel: w417 -> [w432] mode=indexing
              shift-right: [w420] -> w415
              shift-left: w416 -> [w421]
              n168 = Unbundle By Name(w432) -> ("Ch Name"=w424:string, "Position before move (Pulses)"=w431:dbl, "Demanded Position (Pulses)"=w430:dbl, "Minimum Pulses to Move"=w418:dbl, "Pulse Position"=w429:dbl, "Indexer Status Ready?"=w428:bool, "Axis Finished?"=w427:bool, "Limit Switch Valid?"=w419:bool)
              n169 = Build Array(w431, w430, w418, w429) -> (w425:dbl[])
              n170 = Build Array(w428, w427, w419) -> (w426:bool[])
              n171 = Number To Decimal String(number=w425) -> (decimal integer string=w423:string[])  [unwired: 1 out]
              n172 = for {
                tunnel: w426 -> [w434] mode=indexing
                tunnel: [w433] -> w422 mode=indexing
                n173 = Select(t="TRUE", s=w434, f="FALSE") -> (s? t:f=w433:string)
              }
              n174 = Build Array (concatenate)(w421, w424, w423, w422) -> (w420:string[])
            }
          }
          frame #2 {
            n175 = for {
              shift-right: [w446] -> w439
              shift-left: "\r\n" -> [w447]
              tunnel: w442 -> [w445] mode=indexing
              n176 = Concatenate Strings(w447, w445, "\t") -> (w446:string)
            }
            n177 = local read "Log File"() -> (w440:path)
            n178 = local read "Server copy Location"() -> (w438:path)
            n179 = call "Write_File_Simple.vi"("append to file? (new file:F)"=TRUE, "character string"=w439, "file path"=w440) -> ("file path Out"=w437:path)  [unwired: 1 out]
            n180 = call "Updated_File_Copy.vi"("Target Path"=w438, "Source Path"=w437) -> ()  [unwired: 2 out]
          }
        }
      }
    }
  }
